vi "FaultLogger.vi"(10 "Period":i64, 11 "FaultDevRef":T1) -> ()   [LabVIEW 2016]
uses:
  Fault_Fifos.ctl
  Faults.ctl
  <vilib>/Platform/TimedLoop/XDataNode/timing_clust.ctl
  <vilib>/Platform/TimedLoop/XDataNode/nitl_modes.ctl
  <vilib>/Platform/TimedLoop/XDataNode/wakeup.ctl
  Fault_Cluster.ctl
  <vilib>/platform/TimedLoop/XDataNode/XDataNode.xnode
  <vilib>/Platform/TimedLoop/XDataNode/XDNodeRunTimeDep.lvlib
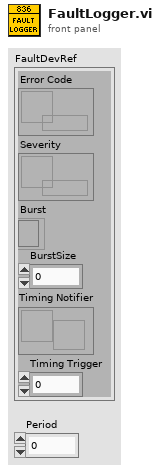
[diagram p1: front panel]
types:
  T1 = typedef "Fault_Fifos.ctl" = cluster{"Error Code":refnum<k33>, "Severity":refnum<k33>, "Burst":refnum<k4>, "BurstSize":u32, "Timing Notifier":refnum<notifier>, "Timing Trigger":u16}
  T2 = typedef "Fault_Cluster.ctl" = cluster{"Error Code":T3, "Severity":u32, "Message":string, "Origin":string}
  T3 = typedef "Faults.ctl" = enum16{"Boiler Target Lost", "Gerar Target Lost", "Body IMU Fault", "Turret IMU Fault"}
  T4 = typedef "XDNodeRunTimeDep.lvlib/timing_clust.ctl" = cluster{"Expected End [f-1]":u64, "Actual End [f-1]":u64, "Finished Late? [f-1]":bool, "Expected End [i-1]":u64, "Actual End [i-1]":u64, "Finished Late? [i-1]":bool, "Expected Start [i]":u64, "Actual Start [i]":u64, "Expected Start [f]":u64, "Actual Start [f]":u64, "Source Name":string, "Structure Name":string, "Period":i64, "Deadline":i64, "Offset":i64, "Start":i64, "Priority":i32, "Timeout":i32, "Mode":T5, "Wakeup Reason":T6, "Error":errorcluster, "Source Type":string, "Secondary Source Type":string, "Global End Time":u64, "Global Start Time":u64, "Frame Duration":u64, "Iteration Duration":u64, "Assigned CPU":i32, "I/O Scan Engine Mode":u32}
  T5 = typedef "XDNodeRunTimeDep.lvlib/nitl_modes.ctl" = enum32{"No Change", "Process missed periods, maintain original phase", "Discard missed periods, maintain original phase", "Process missed periods, ignore original phase", "Discard missed periods, ignore original phase"}
  T6 = typedef "XDNodeRunTimeDep.lvlib/wakeup.ctl" = enum32{"Normal", "Aborted", "Asynchronous wakeup", "Timing source error", "Timed loop error", "Timeout"}
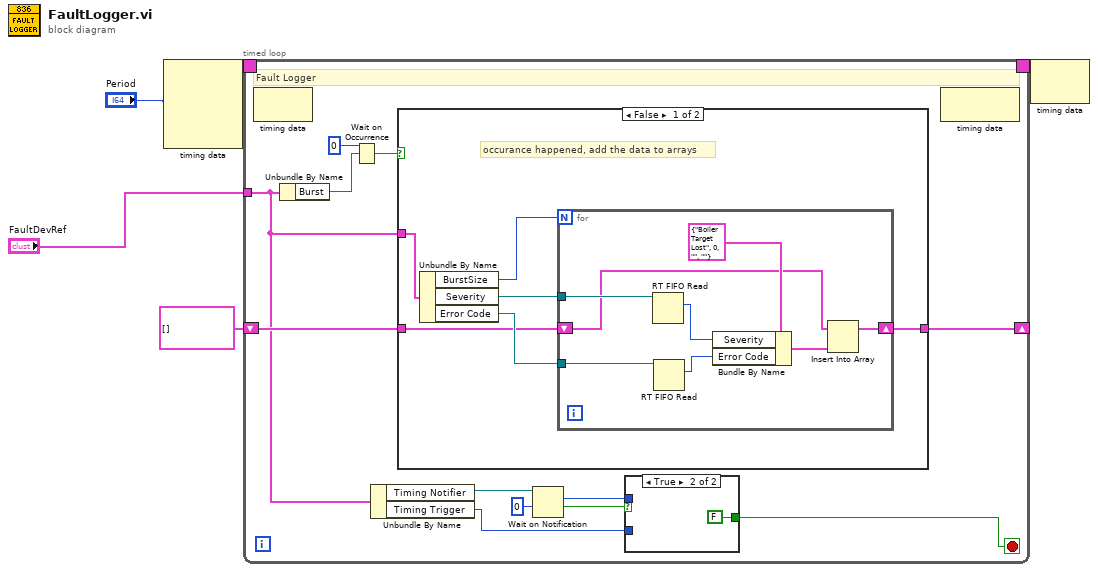
[diagram p0: block diagram]
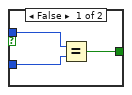
[diagram p2: hidden frame]
diagram:
  n1 = node-c288("Period") -> (w5:T4)  [unwired: 3 in]
  n2 = timed-loop {
    timing: w5 -> [_]
    timing-out: [_] -> w4
    tunnel: "FaultDevRef" -> [w12]
    shift-right: [w14] -> _
    shift-left: T2[] [] -> [w13]
    stop <- w6 stop-if-true
    # "Fault Logger"
    n3 = node-c288() -> ()  [unwired: 1 in, 1 out]
    n4 = Unbundle By Name(w12) -> ("Burst"=w16:refnum<k4>)
    n5 = Wait on Occurrence(2:w16, 3:0 ("ms timeout (-1)")) -> (0:w15:bool)  [unwired: 1 in]
    n6 = Unbundle By Name(w12) -> ("Timing Notifier"=w11:refnum<notifier>, "Timing Trigger"=w7:u16)
    n7 = case shown="False" w15 {
      tunnel: w12 -> [w27 _]
      tunnel: [w23 w36] -> w14
      tunnel: w13 -> [w22 w36]
      frame False {
        # "occurance happened, add the data to arrays"
        n8 = Unbundle By Name(w27) -> ("BurstSize"=w26:u32, "Severity"=w25:refnum<k33>, "Error Code"=w24:refnum<k33>)
        n9 = for {
          N: w26 -> [_]
          tunnel: w25 -> [w35]
          tunnel: w24 -> [w34]
          shift-right: [w29] -> w23
          shift-left: w22 -> [w28]
          n10 = RT FIFO Read(0:w35) -> (9:w32:u32)  [unwired: 3 in, 4 out]
          n11 = RT FIFO Read(0:w34) -> (9:w31:T3)  [unwired: 3 in, 4 out]
          n12 = Bundle By Name(cluster=T2 {"Error Code"=enum."Boiler Target Lost", "Severity"=0, "Message"="", "Origin"=""} ("Fault"), "Severity"=w32, "Error Code"=w31) -> (w30:T2)
          n13 = Insert Into Array(array=w28, new element=w30) -> (w29:T2[])  [unwired: 1 in]
        }
      }
      frame True {
        # "get occurance timed out, therefore no data to log"
      }
    }
    n14 = Wait on Notification(notifier=w11, timeout in ms (-1)=0) -> (notification=w8:u16, timed out?=w9:bool)  [unwired: 2 in, 2 out]
    n15 = case shown="True" w9 {
      tunnel: w8 -> [w19 _]
      tunnel: w7 -> [w20 _]
      tunnel: [w18 FALSE] -> w6
      frame False {
        n16 = Equal?(x=w19, y=w20) -> (x = y?=w18:bool)
      }
      frame True {
      }
    }
    n17 = node-c288() -> ()  [unwired: 1 in, 1 out]
  }
  n18 = node-c288(w4) -> ()  [unwired: 1 out]
